vi "sub_padIQWF.vi"(1 "Repeat":i32, 2 "input complex waveform":cluster{"t0":dbl, "dt":dbl, "Y":cdb[]}, 3 "Packet Pad \n[samples]":i32) -> (0 "output complex waveform":cluster{"t0":dbl, "dt":dbl, "Y":cdb[]})   [LabVIEW 2022 SP3]
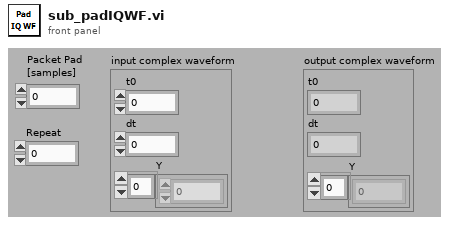
[diagram p1: front panel]
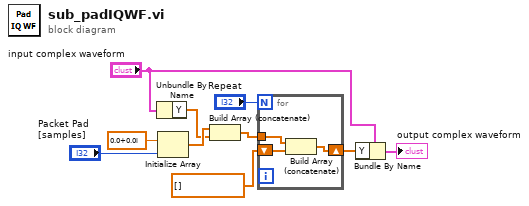
[diagram p0: block diagram]
diagram:
  n1 = Unbundle By Name("input complex waveform") -> ("Y"=w5:cdb[])
  n2 = Initialize Array(cdb 0.0+0.0i ("element"), "Packet Pad \n[samples]") -> (w7:cdb[])
  n3 = Build Array (concatenate)(w7, w5) -> (w3:cdb[])
  n4 = for {
    N: "Repeat" -> [_]
    shift-right: [w11] -> w1
    shift-left: cdb[] [] ("appended array") -> [w13]
    tunnel: w3 -> [w12]
    n5 = Build Array (concatenate)(w12, w13) -> (w11:cdb[])
  }
  n6 = Bundle By Name(cluster="input complex waveform", "Y"=w1) -> (→"output complex waveform":cluster{"t0":dbl, "dt":dbl, "Y":cdb[]})
